vi "Anzeige.vi"(11 "Anzeigeref.":refnum<vi>[](array[refnum])) -> ()   [LabVIEW 2020, in "EPA 1065.lvlib" / "ARN Test 1065-305.lvlib"]
uses:
  ARN Test 1065-305.lvlib
  Aktion FGV ARN Daten.ctl
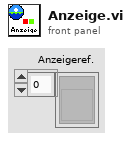
[diagram p1: front panel]
types:
  T1 = typedef "EPA 1065.lvlib/ARN Test 1065-305.lvlib/Aktion FGV ARN Daten.ctl" = enum16{"Lesen", "laden", "speichern", "SNR Info", "Rohdaten", "Rohdaten löschen", "Zeitstempel", "SNR Ergebnis"}
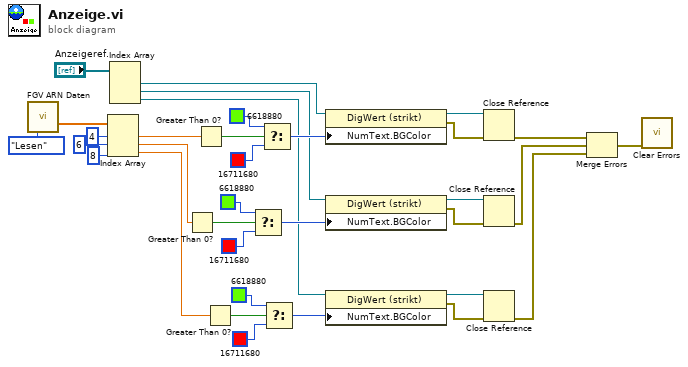
[diagram p0: block diagram]
diagram:
  n1 = call "FGV ARN Daten.vi"("Aktion"=Aktion_FGV_ARN_Daten."Lesen") -> ("SNR Ergebnis"=w33:sgl[])  [unwired: 9 in, 5 out]
  n2 = Index Array(array=w33, index #1=4 ("Index"), index #2=6 ("Index"), index #3=8 ("Index")) -> (element #1=w27:sgl, element #2=w16:sgl, element #3=w15:sgl)
  n3 = Index Array(array="Anzeigeref.") -> (element #1=w31:refnum<vi>, element #2=w13:refnum<vi>, element #3=w11:refnum<vi>)  [unwired: 3 in]
  n4 = Greater Than 0?(x=w16) -> (x > 0?=w22:bool)
  n5 = Greater Than 0?(x=w27) -> (x > 0?=w30:bool)
  n6 = Greater Than 0?(x=w15) -> (x > 0?=w21:bool)
  n7 = Select(t=u32 6618880, s=w22, f=u32 16711680) -> (s? t:f=w14:u32)
  n8 = Select(t=u32 6618880, s=w30, f=u32 16711680) -> (s? t:f=w25:u32)
  n9 = Select(t=u32 6618880, s=w21, f=u32 16711680) -> (s? t:f=w12:u32)
  n10 = property class="DigWert (strikt)"(reference=w31, "NumText.BGColor"=w25) -> (reference out=w10:refnum<vi>, error out=w7:errorcluster)  [unwired: 1 in]
  n11 = property class="DigWert (strikt)"(reference=w13, "NumText.BGColor"=w14) -> (reference out=w9:refnum<vi>, error out=w6:errorcluster)  [unwired: 1 in]
  n12 = property class="DigWert (strikt)"(reference=w11, "NumText.BGColor"=w12) -> (reference out=w8:refnum<vi>, error out=w5:errorcluster)  [unwired: 1 in]
  n13 = Close Reference(reference=w10, error in (no error)=w7) -> (error out=w4:errorcluster)
  n14 = Close Reference(reference=w9, error in (no error)=w6) -> (error out=w3:errorcluster)
  n15 = Close Reference(reference=w8, error in (no error)=w5) -> (error out=w2:errorcluster)
  n16 = Merge Errors(w4, w3, w2) -> (w1:errorcluster)
  n17 = call <vilib>:"Clear Errors.vi"("error in (no error)"=w1) -> ()  [unwired: 5 in, 2 out]
